vi "configure.vi"(8 "error in (no error)":errorcluster, 9 "Serial Message Parameters":T1={"Byte Count"=200, "Enable Termination Character"=FALSE, "Termination Char"=200} {"Termination Char" format="%x"}, 10 "Protocol Parameters":T2={"VISA resource name"="", "Baud Rate"=9600, "Data Bits"=8, "Parity"=enum."None", "Flow Control"=0, "Stop Bits"=10, "Timeout (ms)"=10000} {"Stop Bits" items=["1.0"=10, "1.5"=15, "2.0"=20]; "Flow Control" items=["None", "XON/XOFF", "RTS/CTS", "XON/XOFF & RTS/CTS", "DTR/DSR", "XON/XOFF & DTR/DSR"]; "Data Bits" min=5 max=8 step=1}, 11 "SerialReal in":refnum<class "SerialReal.lvclass">) -> (0 "error out":errorcluster, 3 "SerialReal out":refnum<class "SerialReal.lvclass">)   [LabVIEW 2013, in "SerialProtocols.lvlib" / "SerialReal.lvclass"]
uses:
  <userlib>/Common/SerialProtocols/SerialProtocol/SerialReal/SerialReal.lvclass
  <userlib>/Common/SerialProtocols/Configuration/ProtocolParameters.ctl
  <userlib>/Common/SerialProtocols/Configuration/SerialMessageParameters.ctl
  <userlib>/Common/SerialProtocols/SerialProtocol/SerialReal/SerialReal.lvclass/SerialReal.ctl
  <vilib>/Instr/_visa.llb/VISA Configure Serial Port (Instr).vi
  <userlib>/Common/SerialProtocols/SerialProtocols.lvlib
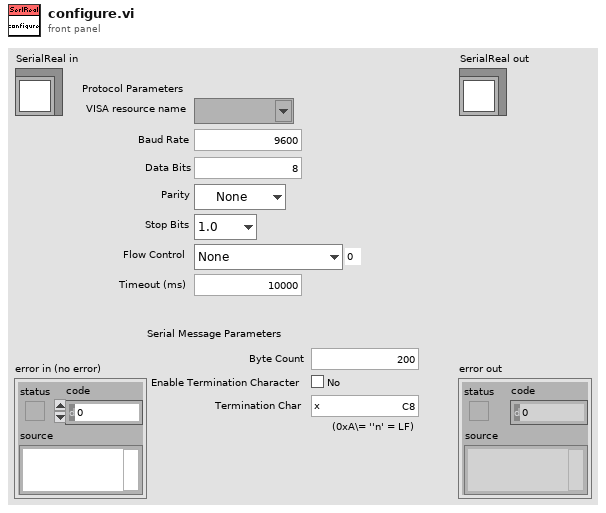
[diagram p1: front panel]
types:
  T1 = typedef "SerialProtocols.lvlib/SerialMessageParameters.ctl" = cluster{"Byte Count":u32, "Enable Termination Character":bool, "Termination Char":u8}
  T2 = typedef "SerialProtocols.lvlib/ProtocolParameters.ctl" = cluster{"VISA resource name":refnum<visa-resource-name>, "Baud Rate":u32, "Data Bits":u16, "Parity":enum16{"None", "Odd", "Even", "Mark", "Space"}, "Flow Control":u16, "Stop Bits":u16, "Timeout (ms)":u32}
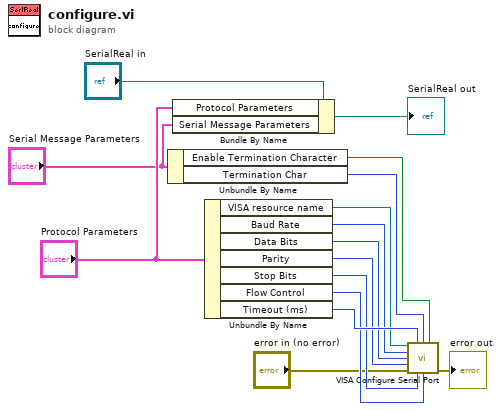
[diagram p0: block diagram]
diagram:
  n1 = Unbundle By Name("Serial Message Parameters") -> ("Enable Termination Character"=w3:bool, "Termination Char"=w2:u8)
  n2 = Bundle By Name(cluster="SerialReal in", "Protocol Parameters"="Protocol Parameters", "Serial Message Parameters"="Serial Message Parameters") -> (→"SerialReal out":refnum<class "SerialReal.lvclass">)
  n3 = Unbundle By Name("Protocol Parameters") -> ("VISA resource name"=w14:refnum<visa-resource-name>, "Baud Rate"=w13:u32, "Data Bits"=w12:u16, "Parity"=w11:enum16{"None", "Odd", "Even", "Mark", "Space"}, "Stop Bits"=w10:u16, "Flow Control"=w9:u16, "Timeout (ms)"=w15:u32)
  n4 = call-poly "VISA Configure Serial Port"("VISA resource name"=w14, "timeout (10sec)"=w15, "termination char\n(0xA = '\\n' = LF)"=w2, "Enable Termination\nChar (T)"=w3, "baud rate (9600)"=w13, "data bits (8)"=w12, "parity (0:none)"=w11, "error in (no error)"="error in (no error)", "stop bits (10: 1 bit)"=w10, "flow control (0:none)"=w9) -> ("error out"=→"error out":errorcluster)  [unwired: 4 in, 1 out]
